vi "Read size 2 Input Register.vi"(8 "error in":errorcluster, 9 "data address":i32, 10 "device ID":u8, 11 "VISA resource name":refnum<visa-resource-name>) -> (0 "error out":errorcluster, 2 "Meter reading":sgl, 3 "VISA resource name out":refnum<visa-resource-name>, 5 "device ID out":i32)   [LabVIEW 2015]
doc: "The master uses this VI to read the slaves input registers. This corresponds to a public function code of 4 in the MODBUS protocol."
uses:
  MB Modbus Command.ctl
panel:
  out "Exception Code":u8 format="%.0x"
  in  "Timeout":u32=120
  # "80 mS causes timeout"
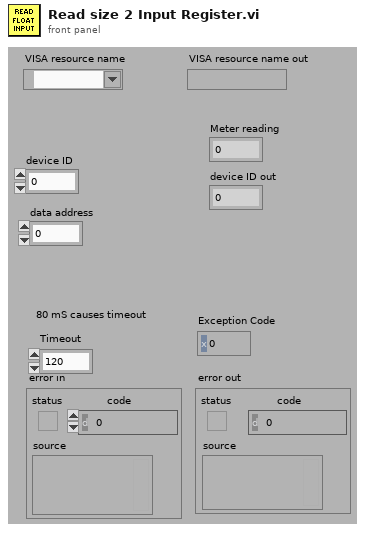
[diagram p1: front panel]
types:
  T1 = typedef "MB Modbus Command.ctl" = cluster{"Function Code":u8, "Starting Address":u16, "Quantity":u16, "Data":u16[], "Discrete":bool[]}
  T2 = cluster{"Mode":enum16{"RTU", "ASCII"}, "device ID":u8}
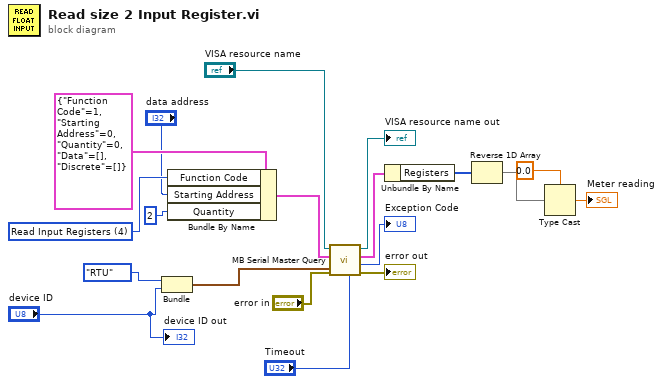
[diagram p0: block diagram]
diagram:
  w16 = u8 4 items=["Read Coils"=1, "Read Discrete Inputs"=2, "Read Holding Registers"=3, "Read Input Registers"=4, "Write Single Coil"=5, "Write Single Register"=6, "Read Exception Status"=7, "Write Multiple Coils"=15, "Write Multiple Registers"=16] ("Function Code")
  n1 = Bundle("Mode"=enum16{"RTU", "ASCII"}."RTU", "device ID"="device ID") -> (w3:T2)  [unwired: 1 in]
  n2 = Bundle By Name(cluster=T1 {"Function Code"=1, "Starting Address"=0, "Quantity"=0, "Data"=[], "Discrete"=[]} ("Modbus Command"), "Function Code"=w16, "Starting Address"="data address", "Quantity"=u16 2) -> (w17:T1)
  n3 = call "MB Serial Master Query.vi"("Timeout"="Timeout", "Serial Parameters"=w3, "error in (no error)"="error in", "Modbus Command"=w17, "VISA resource name"="VISA resource name") -> ("error out"=→"error out":errorcluster, "Exception Code"=→"Exception Code":u8, "Registers"=w9:cluster{"Registers":u16[], "Discrete":bool[]}, "VISA resource name out"=→"VISA resource name out":refnum<visa-resource-name>)  [unwired: 2 in, 1 out]
  n4 = Unbundle By Name(w9) -> ("Registers"=w6:u16[])
  n5 = Reverse 1D Array(array=w6) -> (reversed array=w5:u16[])
  n6 = Type Cast(type=sgl 0.0, x=w5) -> (*(type *) &x=→"Meter reading":sgl)
  "device ID out" <- "device ID"
